vi "List Policy Names.vi"(8 "error in (no error)":errorcluster, 11 "IoT Session in":refnum<class "IoT Session.lvclass">) -> (0 "error out":errorcluster, 2 "Policy Names":string[](array[string]), 3 "IoT Session out":refnum<class "IoT Session.lvclass">)   [LabVIEW 2015, in "NI_AWS_IoT.lvlib" / "IoT Session.lvclass"]
uses:
  IoT Session.lvclass
  Core/HTTP Request/Request Options.ctl
  Core/HTTP Request/Name Value Pair.ctl
  Core/HTTP Request/Region handling.ctl
  Core/HTTP Request/URL formatting.ctl
  Core/HTTP Request/HTTP Request.lvclass
  JSON Parsing/NI_JSON Parsing.lvlib
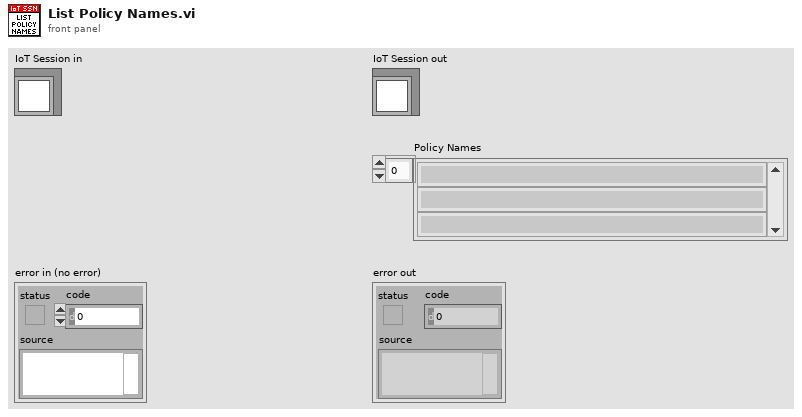
[diagram p1: front panel]
types:
  T1 = typedef "NI_AWS_Core.lvlib/HTTP Request.lvclass/Name Value Pair.ctl" = cluster{"name":string, "value":string}
  T2 = typedef "NI_AWS_Core.lvlib/HTTP Request.lvclass/Request Options.ctl" = cluster{"request headers":T1[], "request parameters":T1[], "request body":string, "region handling":T3, "URL formatting":T4}
  T3 = typedef "NI_AWS_Core.lvlib/HTTP Request.lvclass/Region handling.ctl" = enum16{"use region everywhere", "use region (authentication only)", "use region (URL only)", "ignore region everwhere"}
  T4 = typedef "NI_AWS_Core.lvlib/HTTP Request.lvclass/URL formatting.ctl" = enum16{"region-", "region."}
  T5 = typedef "NI_AWS_Core.lvlib/HTTP Request.lvclass/Response.ctl" = cluster{"Headers":string, "Body":string}
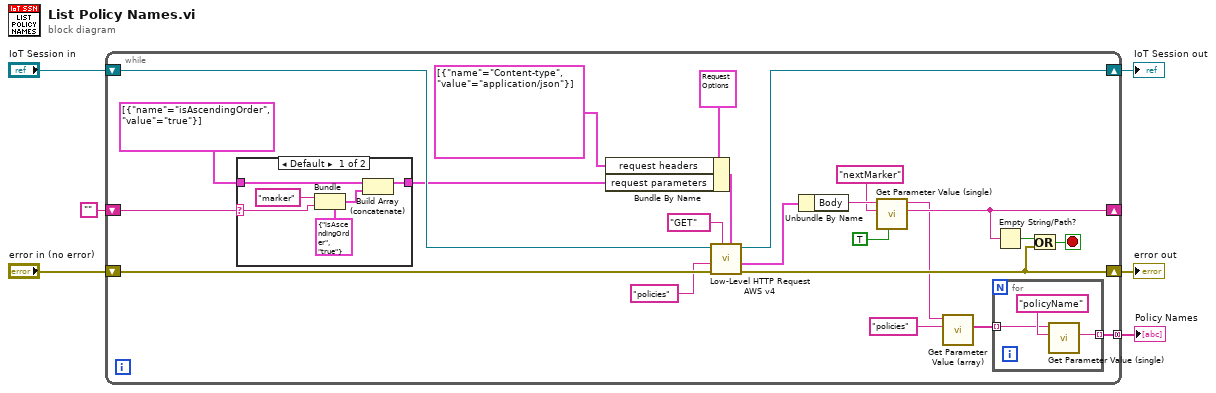
[diagram p0: block diagram]
diagram:
  n1 = while {
    shift-right: [w16] -> w5
    shift-left: "error in (no error)" -> [w26]
    shift-right: [w25] -> w4
    shift-left: "IoT Session in" -> [w24]
    shift-right: [w18] -> _
    shift-left: "" -> [w21]
    tunnel: [w14] -> w1 mode=concatenating
    stop <- w15 stop-if-true
    n2 = case shown="Default" w21 {
      selector: w21 -> [w31 _]
      tunnel: T1[] [{"name"="isAscendingOrder", "value"="true"}] ("request parameters") -> [w35 w36]
      tunnel: [w34 w36] -> w7
      frame Default {
        n3 = Bundle(cluster=T1 {"name"="isAscendingOrder", "value"="true"} ("Name Value Pair"), "name"="marker", "value"=w31) -> (w32:T1)
        n4 = Build Array (concatenate)(w35, w32) -> (w34:T1[])
      }
      frame "" {
      }
    }
    n5 = Bundle By Name(cluster=T2 {"request headers"=[], "request parameters"=[], "request body"="", "region handling"=enum."use region everywhere", "URL formatting"=enum."region."} ("Request Options"), "request headers"=T1[] [{"name"="Content-type", "value"="application/json"}], "request parameters"=w7) -> (w27:T2)
    n6 = call "Low-Level HTTP Request AWS v4.vi"("Request Options"=w27, "HTTP-Verb"="GET", "error in (no error)"=w26, "URL Suffix"="policies" ("string"), "AWS Core in"=w24) -> ("error out"=w16:errorcluster, "Response"=w22:T5, "AWS Core out"=w25:refnum<class "IoT Session.lvclass">)  [unwired: 3 in, 1 out]
    n7 = Unbundle By Name(w22) -> ("Body"=w20:string)
    n8 = call "Get Parameter Value (single).vi"("Clear Null"=TRUE, "Parameter Name"="nextMarker", "JSON"=w20) -> ("Parameter Value"=w18:string, "Remaining JSON"=w13:string)  [unwired: 5 in, 2 out]
    n9 = call "Get Parameter Value (array).vi"("Parameter Name"="policies", "JSON"=w13) -> ("Parameter Values"=w11:string[])  [unwired: 7 in, 2 out]
    n10 = for {
      tunnel: [w37] -> w14 mode=indexing
      tunnel: w11 -> [w38] mode=indexing
      n11 = call "Get Parameter Value (single).vi"("Parameter Name"="policyName", "JSON"=w38) -> ("Parameter Value"=w37:string)  [unwired: 6 in, 3 out]
    }
    n12 = Empty String/Path?(string/path=w18) -> (empty?=w17:bool)
    n13 = Or(x=w17, y=w16) -> (x .or. y?=w15:bool)
  }
  "error out" <- w5
  "IoT Session out" <- w4
  "Policy Names" <- w1
